vi "adam5000-setup-visa.vi"(7 "timeout (10sec)":u32=4000, 8 "error in":errorcluster, 10 "baud rate (19200)":u32=19200, 11 "VISA Refnum in":refnum<visa-resource-name>) -> (0 "error out":errorcluster, 3 "VISA Refnum out":refnum<visa-resource-name>)   [LabVIEW 2020]
uses:
  <vilib>/Instr/_visa.llb/VISA Configure Serial Port (Instr).vi
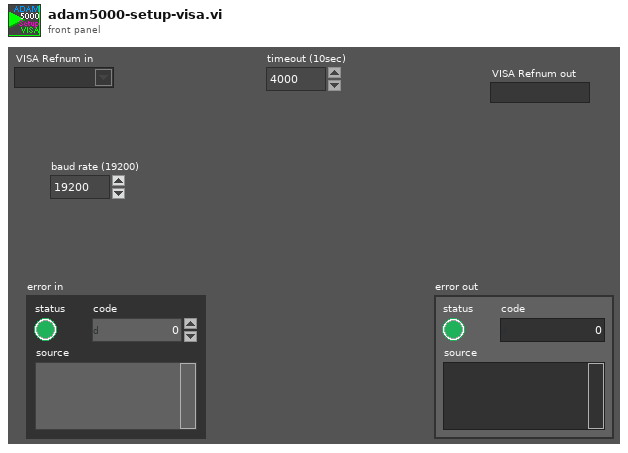
[diagram p1: front panel]
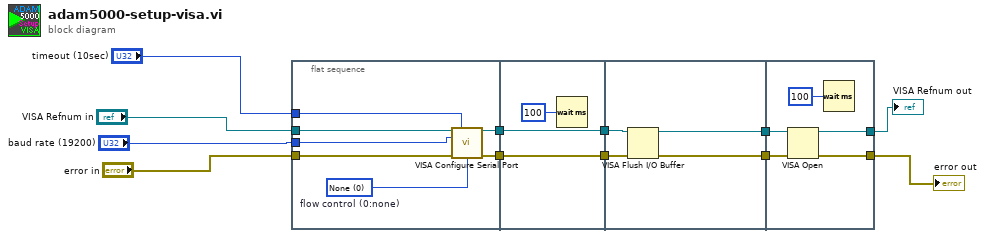
[diagram p0: block diagram]
diagram:
  n1 = flat-sequence {
    tunnel: [w19] -> w12
    tunnel: [w18] -> w11
    tunnel: "VISA Refnum in" -> [w16]
    tunnel: "error in" -> [w15]
    tunnel: "timeout (10sec)" -> [w14]
    tunnel: "baud rate (19200)" -> [w13]
    tunnel: w12 -> [w22]
    tunnel: [w22] -> w10
    tunnel: w11 -> [w21]
    tunnel: [w21] -> w9
    tunnel: w10 -> [w26]
    tunnel: [w24] -> w8
    tunnel: w9 -> [w25]
    tunnel: [w23] -> w7
    tunnel: w8 -> [w30]
    tunnel: w7 -> [w29]
    tunnel: [w28] -> w4
    tunnel: [w27] -> w5
    frame #0 {
      w17 = u16 0 items=["None", "XON/XOFF", "RTS/CTS", "XON/XOFF & RTS/CTS", "DTR/DSR", "XON/XOFF & DTR/DSR"]  # flow control (0:none)
      n2 = call-poly "VISA Configure Serial Port"("VISA resource name"=w16, "timeout (10sec)"=w14, "baud rate (9600)"=w13, "error in (no error)"=w15, "flow control (0:none)"=w17) -> ("VISA resource name out"=w19:refnum<visa-resource-name>, "error out"=w18:errorcluster)  [unwired: 9 in]
    }
    frame #1 {
      n3 = Wait (ms)(milliseconds to wait=u32 100) -> ()  [unwired: 1 out]
    }
    frame #2 {
      n4 = VISA Flush I/O Buffer(VISA resource name=w26, error in (no error)=w25) -> (VISA resource name out=w24:refnum<visa-resource-name>, error out=w23:errorcluster)  [unwired: 1 in]
    }
    frame #3 {
      n5 = VISA Open(error in (no error)=w29, VISA resource name=w30) -> (VISA resource name=w28:refnum<visa-resource-name>, error out=w27:errorcluster)  [unwired: 3 in]
      n6 = Wait (ms)(milliseconds to wait=u32 100) -> ()  [unwired: 1 out]
    }
  }
  "VISA Refnum out" <- w4
  "error out" <- w5
